vi "Create.vi"(5 "FIFO Options":T2, 7 "fifo depths (100)":u32=100, 8 "error in (no error)":errorcluster, 10 "thread settings":T1={"Priority"=100, "Processor"=-2, "ID"=0}, 11 "log file directory":path) -> (0 "error out":errorcluster, 2 "Logging Interface":refnum<class "Logging Interface.lvclass">, 3 "Logging Thread out":refnum<class "Logging Thread.lvclass">)   [LabVIEW 2017, in "DSF Core.lvlib" / "Logging Thread.lvclass"]
uses:
  Logging Thread.lvclass
  C:/Git/DSF/Core/Classes/Thread/Thread.lvclass
  Typedefs/DSF FIFO Options.ctl
  Interface/Logging/Logging Interface.lvclass
  Thread Settings.ctl
  Thread.lvclass/Thread.ctl
  Logging Thread.lvclass/Logging Thread.ctl
  Thread.lvclass
  DSF Core.lvlib
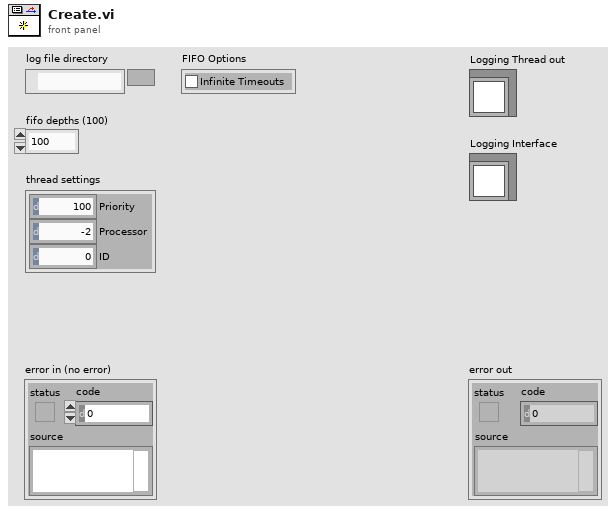
[diagram p1: front panel]
types:
  T1 = typedef "DSF Core.lvlib/Thread.lvclass/Thread Settings.ctl" = cluster{"Priority":u16, "Processor":i32, "ID":i32}
  T2 = typedef "DSF Core.lvlib/DSF FIFO Options.ctl" = cluster{"Infinite Timeouts":bool}
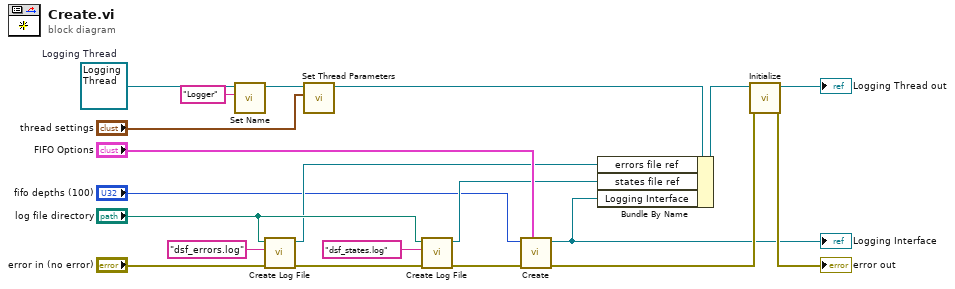
[diagram p0: block diagram]
diagram:
  w8 = refnum<class "Logging Thread.lvclass"> refnum  # Logging Thread
  n1 = call "Set Name.vi"("name"="Logger", "Thread in"=w8) -> ("Thread out"=w7:refnum<class "Logging Thread.lvclass">)  [unwired: 9 in]
  n2 = call "Create Log File.vi"("error in (no error)"="error in (no error)", "log file name"="dsf_errors.log" ("name or relative path"), "log file directory"="log file directory") -> ("error out"=w16:errorcluster, "file refnum"=w10:refnum<file>)  [unwired: 7 in]
  n3 = call "Set Thread Parameters.vi"("thread settings"="thread settings", "Thread in"=w7) -> ("Thread out"=w6:refnum<class "Logging Thread.lvclass">)  [unwired: 9 in]
  n4 = call "Create Log File.vi"("error in (no error)"=w16, "log file name"="dsf_states.log" ("name or relative path"), "log file directory"="log file directory") -> ("error out"=w11:errorcluster, "file refnum"=w15:refnum<file>)  [unwired: 7 in]
  n5 = call "Create.vi"("FIFO Options"="FIFO Options", "error in (no error)"=w11, "fifo/queue depths (10)"="fifo depths (100)") -> ("error out"=w3:errorcluster, "Logging Interface out"=w1:refnum<class "Logging Interface.lvclass">)  [unwired: 7 in]
  "Logging Interface" <- w1
  n6 = Bundle By Name(cluster=w6, "errors file ref"=w10, "states file ref"=w15, "Logging Interface"=w1) -> (w5:refnum<class "Logging Thread.lvclass">)
  n7 = call-dynamic "Initialize.vi"("error in (no error)"=w3, "Thread in"=w5) -> ("error out"=→"error out":errorcluster, "Thread out"=→"Logging Thread out":refnum<class "Logging Thread.lvclass">)  [unwired: 8 in]
